vi "Receive.vi"(8 "error in (no error)":errorcluster, 11 "Fake ILC in":refnum<class "Fake ILC.lvclass">) -> (0 "error out":errorcluster, 2 "Response":string, 3 "Fake ILC out":refnum<class "Fake ILC.lvclass">)   [LabVIEW 2015, in "Fake ILC.lvclass"]
uses:
  Fake ILC.lvclass
  <userlib>/Common/ILC/ILC/ILC.lvclass/ILC.ctl
  Fake ILC.lvclass/Fake ILC.ctl
  <userlib>/Common/ILC/ILC/ILC.lvclass
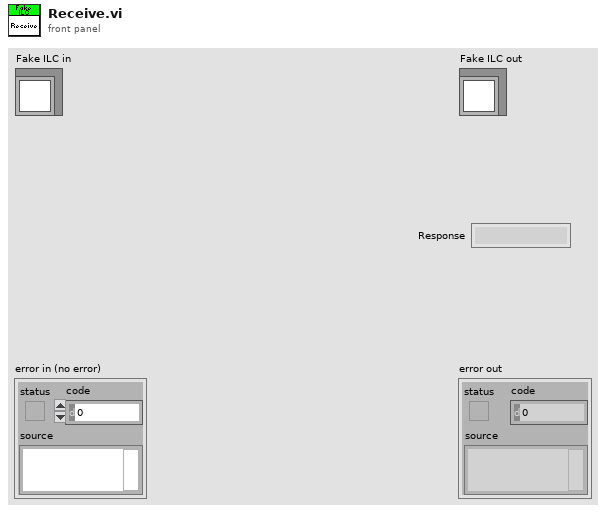
[diagram p1: front panel]
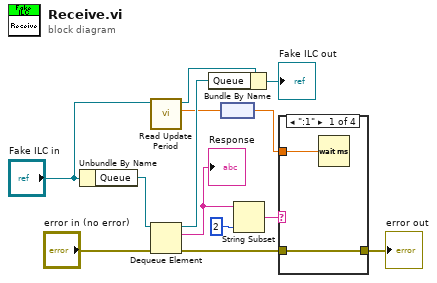
[diagram p0: block diagram]
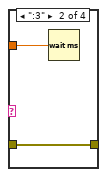
[diagram p2: hidden frame]
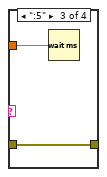
[diagram p3: hidden frame]
diagram:
  n1 = Unbundle By Name("Fake ILC in") -> ("Queue"=w12:refnum<queue>)
  n2 = call <userlib>:"Read Update Period.vi"("ILC in"="Fake ILC in") -> ("Update Period"=w4:dbl[unit], "ILC out"=w5:refnum<class "Fake ILC.lvclass">)  [unwired: 9 in]
  n3 = Dequeue Element(queue=w12, error in (no error)="error in (no error)") -> (queue out=w11:refnum<queue>, element=w8:string, error out=w3:errorcluster)  [unwired: 1 in, 1 out]
  "Response" <- w8
  n4 = Bundle By Name(cluster=w5, "Queue"=w11) -> (→"Fake ILC out":refnum<class "Fake ILC.lvclass">)
  n5 = node(w4) -> (w1:dbl)
  n6 = String Subset(string=w8, length (rest)=2 ("length (rest)")) -> (substring=w7:string)  [unwired: 1 in]
  n7 = case shown="\":1\"" w7 {
    tunnel: w1 -> [w15 w17 w19 _]
    tunnel: w3 -> [w14 w16 w18 w20]
    tunnel: [w14 w16 w18 w20] -> w2
    frame ":1" {
      n8 = Wait (ms)(milliseconds to wait=w15) -> ()  [unwired: 1 out]
    }
    frame ":3" {
      n9 = Wait (ms)(milliseconds to wait=w17) -> ()  [unwired: 1 out]
    }
    frame ":5" {
      n10 = Wait (ms)(milliseconds to wait=w19) -> ()  [unwired: 1 out]
    }
    frame Default {
    }
  }
  "error out" <- w2
